vi "stepTriggerGlobalVars.vi"() -> ()   [LabVIEW 2014]
uses:
  Controls/triggerTypes.ctl
  Controls/selectTrigger.ctl
  Controls/triggerEdge.ctl
panel:
  in  "softwareStepTrigger":bool
  in  "stepTriggerEdge":T1=enum."true-false"
  in  "selectStepTrigger":T2
  in  "step_trig_delay_10ns_ticks":u32
  in  "stepTriggerTypes":T3
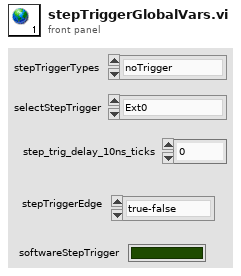
[diagram p1: front panel]
types:
  T1 = typedef "triggerEdge.ctl" = enum8{"either", "false-true", "true-false"}
  T2 = typedef "selectTrigger.ctl" = enum8{"Ext0", "Ext1", "Ext2", "Ext3", "Ext4", "Ext5", "Ext6", "Ext7", "Int0", "Int1", "Int2", "Int3", "Int4", "Int5", "Int6", "Int7"}
  T3 = typedef "triggerTypes.ctl" = enum16{"noTrigger", "singleHitDelay", "singleHit", "software", "sweep"}
diagram:
